vi "Create Display Objects.vi"(8 "Error In":errorcluster, 11 "Display Manager In":refnum<class "Display Manager.lvclass">) -> (0 "Error Out":errorcluster, 3 "Display Manager Out":refnum<class "Display Manager.lvclass">)   [LabVIEW 2019, in "Display Manager.lvclass"]
uses:
  Display Manager.lvclass
  <vilib>/Memosfet/myRIO-Neopixel/RT/Display/Public/Controls/RGB Gains.ctl
  Accessors/Display Mode/Get Display Mode.vi
  Accessors/Display/Get Display.vi
  <vilib>/Memosfet/myRIO-Neopixel/RT/Display/Display.lvclass
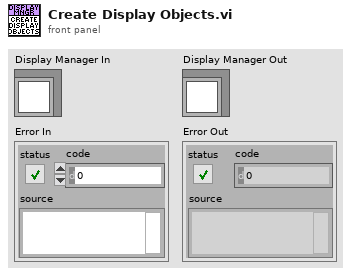
[diagram p1: front panel]
types:
  T1 = typedef "Display.lvclass/RGB Gains.ctl" = cluster{"Red":sgl, "Green":sgl, "Blue":sgl}
  T2 = typedef "Display Manager.lvclass/Display Mode.ctl" = enum16{"Dashboard", "Audio Analyzer"}
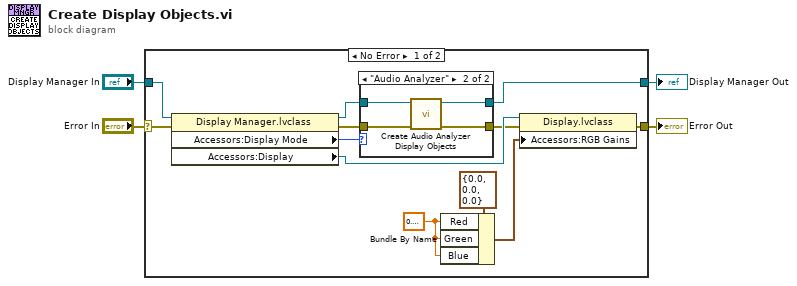
[diagram p0: block diagram]
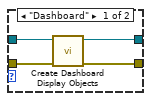
[diagram p2: hidden frame]
diagram:
  n1 = case shown="No Error" "Error In" {
    selector: "Error In" -> [w15 w26]
    tunnel: [w5 w26] -> w3
    tunnel: "Display Manager In" -> [w16 w25]
    tunnel: [w13 w25] -> w1
    frame No Error {
      w7 = sgl 0.1 ("Red")
      n2 = property class="Display Manager.lvclass"(reference=w16, error in=w15) -> (reference out=w11:refnum<class "Display Manager.lvclass">, error out=w12:errorcluster, "Accessors:Display Mode"=w14:T2, "Accessors:Display"=w10:refnum<class "Display.lvclass">)
      n3 = case shown="\"Audio Analyzer\"" w14 {
        tunnel: [w18 w22] -> w13
        tunnel: w12 -> [w20 w23]
        tunnel: w11 -> [w19 w24]
        tunnel: [w17 w21] -> w9
        frame "Dashboard" {
          n4 = call "Create Dashboard Display Objects.vi"("Error In"=w20, "Display Manager In"=w19) -> ("Error Out"=w17:errorcluster, "Display Manager Out"=w18:refnum<class "Display Manager.lvclass">)  [unwired: 8 in]
        }
        frame "Audio Analyzer" {
          n5 = call "Create Audio Analyzer Display Objects.vi"("Error In"=w23, "Display Manager In"=w24) -> ("Error Out"=w21:errorcluster, "Display Manager Out"=w22:refnum<class "Display Manager.lvclass">)  [unwired: 8 in]
        }
      }
      n6 = Bundle By Name(cluster=T1 {"Red"=0.0, "Green"=0.0, "Blue"=0.0} ("RGB Gains"), "Red"=w7, "Green"=w7, "Blue"=w7) -> (w8:T1)
      n7 = property class="Display.lvclass"(reference=w10, error in=w9, "Accessors:RGB Gains"=w8) -> (error out=w5:errorcluster)  [unwired: 1 out]
    }
    frame Error {
    }
  }
  "Display Manager Out" <- w1
  "Error Out" <- w3
